vi "Load processed data.vi"(6 "EXE distribution?":bool=TRUE, 8 "error in (not an error)":errorcluster, 9 "Prompt":string="Load intermedia data file", 10 "start path":path, 11 "file path":path) -> (0 "error out":errorcluster, 1 "parameters":cluster{"sample rate":sgl, "pulses/rev":i32} {"sample rate" format="%.2f"}, 2 "speed profile":T2 {"speed [RPM]" format="%.2f"; "time [s]" format="%.2f"}, 3 "S&V samples":dbl[](array[numeric]) format="%.2f", 4 "window info":T1={"window type"=3, "window length"=2048} {"window type" items=["None"=0, "Hanning"=1, "Hamming"=2, "Blackman-Harris"=3, "Exact Blackman"=4, "Blackman"=5, "Flat Top"=6, "4 Term B-Harris"=7, "7 Term B-Harris"=8, "Low Sidelobe"=9, "Gaussian"=62]; "window length" min=0}, 5 "lables":cluster{"tach lable":string, "S&V lable":string}, 7 "file path out":path)   [LabVIEW 2017]
uses:
  <vilib>/addons/Sound and Vibration/Order Analysis/Tach Process/SubVIs/speed profile.ctl
  <vilib>/addons/Sound and Vibration/Order Analysis/Ref Gabor Order Tracking/window information.ctl
  <vilib>/addons/Sound and Vibration/Order Analysis/Gabor Order Tracking/SoundVib_Gabor.lvlib
  <vilib>/addons/Sound and Vibration/Order Analysis/Tach Process/SoundVib_TachProcess.lvlib
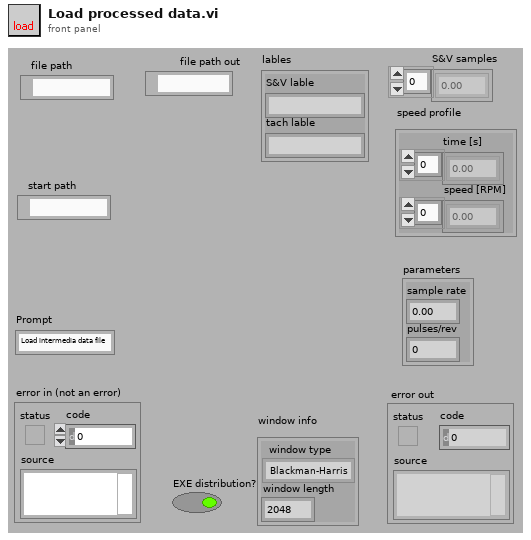
[diagram p1: front panel]
types:
  T1 = typedef "SoundVib_Gabor.lvlib/window information.ctl" = cluster{"window type":u32, "window length":i32}
  T2 = typedef "SoundVib_TachProcess.lvlib/speed profile.ctl" = cluster{"time [s]":dbl[], "speed [RPM]":dbl[]}
  T3 = cluster{"lables":cluster{"tach lable":string, "S&V lable":string}, "S&V samples":dbl[], "speed profile":cluster{"time [s]":dbl[], "speed [rpm]":dbl[]}, "parameters":cluster{"sample rate":sgl, "pulses/rev":i32}, "window info":cluster{"window type":enum32{"Hanning", "Hamming", "Blackman", "Gaussian"}, "window length":i32}}[]
  T4 = cluster{"lables":cluster{"tach lable":string, "S&V lable":string}, "S&V samples":dbl[], "speed profile":cluster{"time [s]":dbl[], "speed [rpm]":dbl[]}, "parameters":cluster{"sample rate":sgl, "pulses/rev":i32}, "window info":cluster{"window type":enum32{"Hanning", "Hamming", "Blackman", "Gaussian"}, "window length":i32}}
  T5 = cluster{"window type":enum32{"Hanning", "Hamming", "Blackman", "Gaussian"}, "window length":i32}
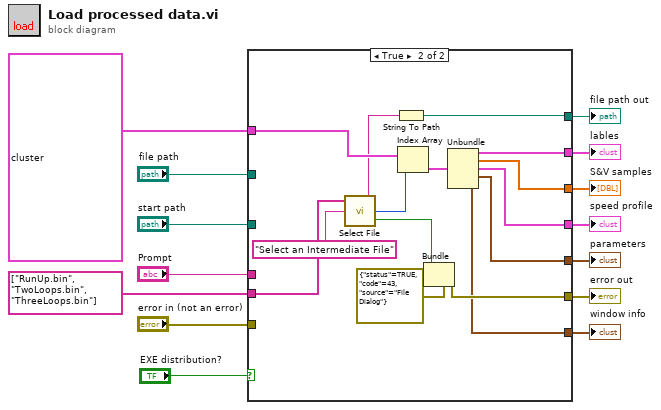
[diagram p0: block diagram]
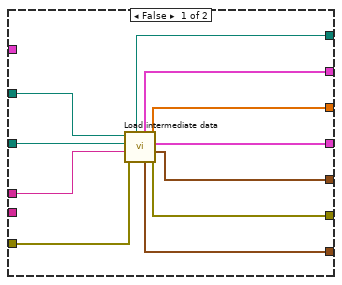
[diagram p2: hidden frame]
diagram:
  n1 = case shown="True" "EXE distribution?" {
    tunnel: [w25 w29] -> w14
    tunnel: [w24 w35] -> w13
    tunnel: [w23 w32] -> w12
    tunnel: [w22 w34] -> w11
    tunnel: [w21 w33] -> w10
    tunnel: [w20 w31] -> w9
    tunnel: [w19 w37] -> w8
    tunnel: "file path" -> [w18 _]
    tunnel: "start path" -> [w17 _]
    tunnel: "Prompt" -> [w16 _]
    tunnel: "error in (not an error)" -> [w15 _]
    tunnel: T3 [{"lables"={"tach lable"="tacho (V)", "S&V lable"="acc H (m/s^2)"}, "S&V samples"=array[55296 elements], "speed profile"={"time [s]"=array[1418 elements], "speed [rpm]"=array[1418 elements]}, "parameters"={"sample rate"=4000.0, "pulses/rev"=2}, "window info"={"window type"=enum."Gaussian", "window length"=2048}}, {"lables"={"tach lable"="Tach (V)", "S&V lable"="Acc Y (g)"}, "S&V samples"=array[73728 elements], "speed profile"={"time [s]"=array[1257 elements], "speed [rpm]"=array[1257 elements]}, "parameters"={"sample rate"=5000.0, "pulses/rev"=2}, "window info"={"window type"=enum."Gaussian", "window length"=2048}}, {"lables"={"tach lable"="Tach (V)", "S&V lable"="Acc X (g)"}, "S&V samples"=array[73728 elements], "speed profile"={"time [s]"=array[1212 elements], "speed [rpm]"=array[1212 elements]}, "parameters"={"sample rate"=5000.0, "pulses/rev"=2}, "window info"={"window type"=enum."Gaussian", "window length"=1024}}] ("Array") -> [_ w39]
    tunnel: string[] ["RunUp.bin", "TwoLoops.bin", "ThreeLoops.bin"] ("Item Names") -> [_ w27]
    frame False {
      n2 = call <vilib>:"Load intermediate data.vi"("error in (not an error)"=w15, "Prompt"=w16, "start path"=w17, "file path"=w18) -> ("error out"=w19:errorcluster, "parameters"=w23:cluster{"sample rate":sgl, "pulses/rev":i32}, "speed profile"=w21:T2, "S&V samples"=w22:dbl[], "window info"=w20:T1, "lables"=w24:cluster{"tach lable":string, "S&V lable":string}, "file path out"=w25:path)  [unwired: 1 in]
    }
    frame True {
      n3 = call <vilib>:"Select File.vi"("prompt"="Select an Intermediate File", "file names"=w27) -> ("canceled"=w38:bool, "index"=w40:i32, "file name"=w30:string)  [unwired: 1 in]
      n4 = String To Path(string=w30) -> (path=w29:path)
      n5 = Index Array(array=w39, index=w40) -> (element=w36:T4)
      n6 = Bundle(cluster=errorcluster {"status"=TRUE, "code"=43, "source"="File Dialog"} ("error out"), "status"=w38) -> (w37:errorcluster)  [unwired: 2 in]
      n7 = Unbundle(w36) -> ("lables"=w35:cluster{"tach lable":string, "S&V lable":string}, "S&V samples"=w34:dbl[], "speed profile"=w33:cluster{"time [s]":dbl[], "speed [rpm]":dbl[]}, "parameters"=w32:cluster{"sample rate":sgl, "pulses/rev":i32}, "window info"=w31:T5)
    }
  }
  "S&V samples" <- w11
  "speed profile" <- w10
  "window info" <- w9
  "error out" <- w8
  "file path out" <- w14
  "parameters" <- w12
  "lables" <- w13
